vi "Window Memory write - Target.vi"(11 "Hanning window":bool=TRUE) -> ()   [LabVIEW 2014]
uses:
  <vilib>/rvi/Emulation/niFpgaGetClockAttributes.vi
  <vilib>/rvi/Emulation/niFpgaSctlEmulationGetInTimedLoop.vi
  <vilib>/rvi/Emulation/niFpgaEmulationReportErrorSimple.vi
  <vilib>/rvi/Memory/Memory_Emulation/nirvimemoryFastEmulation.vi
  <vilib>/rvi/Memory/Memory_Emulation/nirvimemoryEmulation.vi
  <vilib>/rvi/Emulation/niFpgaEmulationIsFPGAContextNoSignature.vi
  <vilib>/rvi/DataTransferAndStorage/Container/Common/niFpgaContainerGetUniqueNameForEmu.vi
  <vilib>/rvi/Emulation/niFpgaProcessEmulError.vi
  <vilib>/rvi/errors/nirviReportUnexpectedCaseInternalError (U32).vi
  <vilib>/rvi/Emulation/niFpgaCriticalErrorInLSC.vi
  <vilib>/rvi/DataTransferAndStorage/Container/XNode/niFpgaContainer.xnode
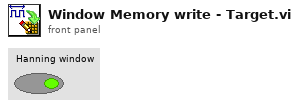
[diagram p1: front panel]
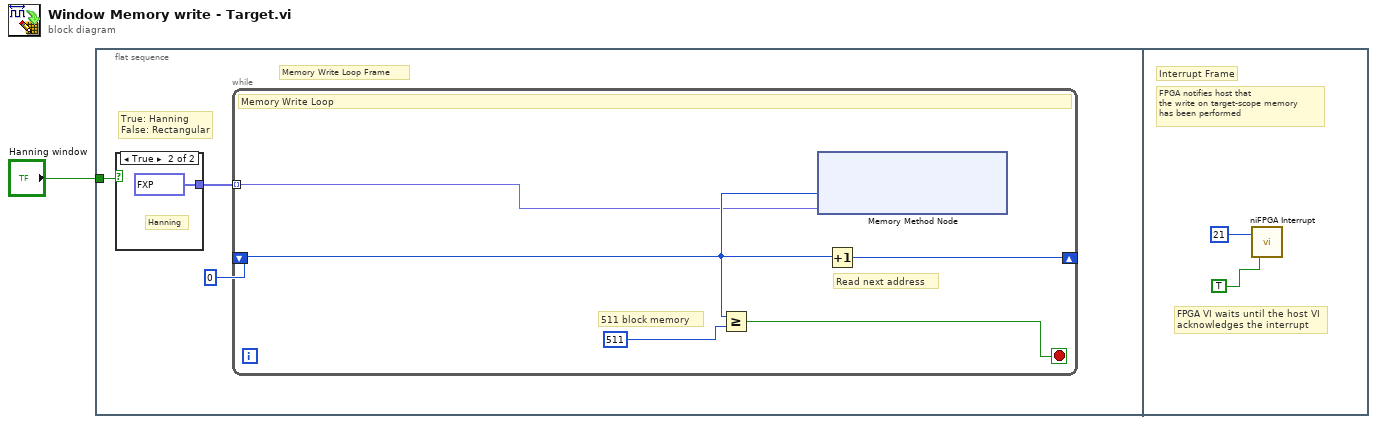
[diagram p0: block diagram]
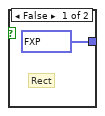
[diagram p2: hidden frame]
diagram:
  n1 = flat-sequence {
    tunnel: "Hanning window" -> [w3]
    frame #0 {
      # "True: Hanning\nFalse: Rectangular"
      # "Memory Write Loop Frame"
      n2 = case shown="True" w3 {
        tunnel: [fxp<+,8,1>[] [1.0, 1.0, 1.0, 1.0, 1.0, 1.0, 1.0, 1.0, 1.0, 1.0, 1.0, 1.0, 1.0, 1.0, 1.0, 1.0, 1.0, 1.0, 1.0, 1.0, 1.0, 1.0, 1.0, 1.0, 1.0, 1.0, 1.0, 1.0, 1.0, 1.0, 1.0, 1.0, 1.0, 1.0, 1.0, 1.0, 1.0, 1.0, 1.0, 1.0, 1.0, 1.0, 1.0, 1.0, 1.0, 1.0, 1.0, 1.0, 1.0, 1.0, 1.0, 1.0, 1.0, 1.0, 1.0, 1.0, 1.0, 1.0, 1.0, 1.0, 1.0, 1.0, 1.0, 1.0, 1.0, 1.0, 1.0, 1.0, 1.0, 1.0, 1.0, 1.0, 1.0, 1.0, 1.0, 1.0, 1.0, 1.0, 1.0, 1.0, 1.0, 1.0, 1.0, 1.0, 1.0, 1.0, 1.0, 1.0, 1.0, 1.0, 1.0, 1.0, 1.0, 1.0, 1.0, 1.0, 1.0, 1.0, 1.0, 1.0, 1.0, 1.0, 1.0, 1.0, 1.0, 1.0, 1.0, 1.0, 1.0, 1.0, 1.0, 1.0, 1.0, 1.0, 1.0, 1.0, 1.0, 1.0, 1.0, 1.0, 1.0, 1.0, 1.0, 1.0, 1.0, 1.0, 1.0, 1.0, 1.0, 1.0, 1.0, 1.0, 1.0, 1.0, 1.0, 1.0, 1.0, 1.0, 1.0, 1.0, 1.0, 1.0, 1.0, 1.0, 1.0, 1.0, 1.0, 1.0, 1.0, 1.0, 1.0, 1.0, 1.0, 1.0, 1.0, 1.0, 1.0, 1.0, 1.0, 1.0, 1.0, 1.0, 1.0, 1.0, 1.0, 1.0, 1.0, 1.0, 1.0, 1.0, 1.0, 1.0, 1.0, 1.0, 1.0, 1.0, 1.0, 1.0, 1.0, 1.0, 1.0, 1.0, 1.0, 1.0, 1.0, 1.0, 1.0, 1.0, 1.0, 1.0, 1.0, 1.0, 1.0, 1.0, 1.0, 1.0, 1.0, 1.0, 1.0, 1.0, 1.0, 1.0, 1.0, 1.0, 1.0, 1.0, 1.0, 1.0, 1.0, 1.0, 1.0, 1.0, 1.0, 1.0, 1.0, 1.0, 1.0, 1.0, 1.0, 1.0, 1.0, 1.0, 1.0, 1.0, 1.0, 1.0, 1.0, 1.0, 1.0, 1.0, 1.0, 1.0, 1.0, 1.0, 1.0, 1.0, 1.0, 1.0, 1.0, 1.0, 1.0, 1.0, 1.0, 1.0, 1.0, 1.0, 1.0, 1.0, 1.0, 1.0, 1.0, 1.0, 1.0, 1.0, 1.0, 1.0, 1.0, 1.0, 1.0, 1.0, 1.0, 1.0, 1.0, 1.0, 1.0, 1.0, 1.0, 1.0, 1.0, 1.0, 1.0, 1.0, 1.0, 1.0, 1.0, 1.0, 1.0, 1.0, 1.0, 1.0, 1.0, 1.0, 1.0, 1.0, 1.0, 1.0, 1.0, 1.0, 1.0, 1.0, 1.0, 1.0, 1.0, 1.0, 1.0, 1.0, 1.0, 1.0, 1.0, 1.0, 1.0, 1.0, 1.0, 1.0, 1.0, 1.0, 1.0, 1.0, 1.0, 1.0, 1.0, 1.0, 1.0, 1.0, 1.0, 1.0, 1.0, 1.0, 1.0, 1.0, 1.0, 1.0, 1.0, 1.0, 1.0, 1.0, 1.0, 1.0, 1.0, 1.0, 1.0, 1.0, 1.0, 1.0, 1.0, 1.0, 1.0, 1.0, 1.0, 1.0, 1.0, 1.0, 1.0, 1.0, 1.0, 1.0, 1.0, 1.0, 1.0, 1.0, 1.0, 1.0, 1.0, 1.0, 1.0, 1.0, 1.0, 1.0, 1.0, 1.0, 1.0, 1.0, 1.0, 1.0, 1.0, 1.0, 1.0, 1.0, 1.0, 1.0, 1.0, 1.0, 1.0, 1.0, 1.0, 1.0, 1.0, 1.0, 1.0, 1.0, 1.0, 1.0, 1.0, 1.0, 1.0, 1.0, 1.0, 1.0, 1.0, 1.0, 1.0, 1.0, 1.0, 1.0, 1.0, 1.0, 1.0, 1.0, 1.0, 1.0, 1.0, 1.0, 1.0, 1.0, 1.0, 1.0, 1.0, 1.0, 1.0, 1.0, 1.0, 1.0, 1.0, 1.0, 1.0, 1.0, 1.0, 1.0, 1.0, 1.0, 1.0, 1.0, 1.0, 1.0, 1.0, 1.0, 1.0, 1.0, 1.0, 1.0, 1.0, 1.0, 1.0, 1.0, 1.0, 1.0, 1.0, 1.0, 1.0, 1.0, 1.0, 1.0, 1.0, 1.0, 1.0, 1.0, 1.0, 1.0, 1.0, 1.0, 1.0, 1.0, 1.0, 1.0, 1.0, 1.0, 1.0, 1.0, 1.0, 1.0, 1.0, 1.0, 1.0, 1.0, 1.0, 1.0, 1.0, 1.0, 1.0, 1.0, 1.0, 1.0, 1.0, 1.0, 1.0, 1.0, 1.0, 1.0, 1.0, 1.0, 1.0, 1.0, 1.0, 1.0, 1.0, 1.0, 1.0, 1.0, 1.0, 1.0, 1.0, 1.0, 1.0, 1.0, 1.0, 1.0, 1.0, 1.0, 1.0, 1.0, 1.0, 1.0, 1.0, 1.0, 1.0, 1.0, 1.0, 1.0, 1.0, 1.0, 1.0, 1.0] ("Window Array") fxp<+,8,1>[] [0.0, 0.0, 0.0, 0.0, 0.0, 0.0, 0.0, 0.0, 0.0, 0.0, 0.0, 0.0078125, 0.0078125, 0.0078125, 0.0078125, 0.0078125, 0.0078125, 0.0078125, 0.015625, 0.015625, 0.015625, 0.015625, 0.015625, 0.0234375, 0.0234375, 0.0234375, 0.0234375, 0.0234375, 0.03125, 0.03125, 0.03125, 0.0390625, 0.0390625, 0.0390625, 0.0390625, 0.046875, 0.046875, 0.046875, 0.0546875, 0.0546875, 0.0625, 0.0625, 0.0625, 0.0703125, 0.0703125, 0.078125, 0.078125, 0.078125, 0.0859375, 0.0859375, 0.09375, 0.09375, 0.1015625, 0.1015625, 0.109375, 0.109375, 0.1171875, 0.1171875, 0.125, 0.125, 0.1328125, 0.1328125, 0.140625, 0.140625, 0.1484375, 0.1484375, 0.15625, 0.15625, 0.1640625, 0.171875, 0.171875, 0.1796875, 0.1796875, 0.1875, 0.1953125, 0.1953125, 0.203125, 0.2109375, 0.2109375, 0.21875, 0.21875, 0.2265625, 0.234375, 0.234375, 0.2421875, 0.25, 0.25, 0.2578125, 0.265625, 0.2734375, 0.2734375, 0.28125, 0.2890625, 0.2890625, 0.296875, 0.3046875, 0.3125, 0.3125, 0.3203125, 0.328125, 0.328125, 0.3359375, 0.34375, 0.3515625, 0.3515625, 0.359375, 0.3671875, 0.375, 0.375, 0.3828125, 0.390625, 0.3984375, 0.40625, 0.40625, 0.4140625, 0.421875, 0.4296875, 0.4296875, 0.4375, 0.4453125, 0.453125, 0.4609375, 0.4609375, 0.46875, 0.4765625, 0.484375, 0.484375, 0.4921875, 0.5, 0.5078125, 0.515625, 0.515625, 0.5234375, 0.53125, 0.5390625, 0.5390625, 0.546875, 0.5546875, 0.5625, 0.5703125, 0.5703125, 0.578125, 0.5859375, 0.59375, 0.59375, 0.6015625, 0.609375, 0.6171875, 0.625, 0.625, 0.6328125, 0.640625, 0.6484375, 0.6484375, 0.65625, 0.6640625, 0.671875, 0.671875, 0.6796875, 0.6875, 0.6875, 0.6953125, 0.703125, 0.7109375, 0.7109375, 0.71875, 0.7265625, 0.7265625, 0.734375, 0.7421875, 0.75, 0.75, 0.7578125, 0.765625, 0.765625, 0.7734375, 0.78125, 0.78125, 0.7890625, 0.7890625, 0.796875, 0.8046875, 0.8046875, 0.8125, 0.8203125, 0.8203125, 0.828125, 0.828125, 0.8359375, 0.84375, 0.84375, 0.8515625, 0.8515625, 0.859375, 0.859375, 0.8671875, 0.8671875, 0.875, 0.875, 0.8828125, 0.8828125, 0.890625, 0.890625, 0.8984375, 0.8984375, 0.90625, 0.90625, 0.9140625, 0.9140625, 0.921875, 0.921875, 0.921875, 0.9296875, 0.9296875, 0.9375, 0.9375, 0.9375, 0.9453125, 0.9453125, 0.953125, 0.953125, 0.953125, 0.9609375, 0.9609375, 0.9609375, 0.9609375, 0.96875, 0.96875, 0.96875, 0.9765625, 0.9765625, 0.9765625, 0.9765625, 0.9765625, 0.984375, 0.984375, 0.984375, 0.984375, 0.984375, 0.9921875, 0.9921875, 0.9921875, 0.9921875, 0.9921875, 0.9921875, 0.9921875, 1.0, 1.0, 1.0, 1.0, 1.0, 1.0, 1.0, 1.0, 1.0, 1.0, 1.0, 1.0, 1.0, 1.0, 1.0, 1.0, 1.0, 1.0, 1.0, 1.0, 1.0, 0.9921875, 0.9921875, 0.9921875, 0.9921875, 0.9921875, 0.9921875, 0.9921875, 0.984375, 0.984375, 0.984375, 0.984375, 0.984375, 0.9765625, 0.9765625, 0.9765625, 0.9765625, 0.9765625, 0.96875, 0.96875, 0.96875, 0.9609375, 0.9609375, 0.9609375, 0.9609375, 0.953125, 0.953125, 0.953125, 0.9453125, 0.9453125, 0.9375, 0.9375, 0.9375, 0.9296875, 0.9296875, 0.921875, 0.921875, 0.921875, 0.9140625, 0.9140625, 0.90625, 0.90625, 0.8984375, 0.8984375, 0.890625, 0.890625, 0.8828125, 0.8828125, 0.875, 0.875, 0.8671875, 0.8671875, 0.859375, 0.859375, 0.8515625, 0.8515625, 0.84375, 0.84375, 0.8359375, 0.828125, 0.828125, 0.8203125, 0.8203125, 0.8125, 0.8046875, 0.8046875, 0.796875, 0.7890625, 0.7890625, 0.78125, 0.78125, 0.7734375, 0.765625, 0.765625, 0.7578125, 0.75, 0.75, 0.7421875, 0.734375, 0.7265625, 0.7265625, 0.71875, 0.7109375, 0.7109375, 0.703125, 0.6953125, 0.6875, 0.6875, 0.6796875, 0.671875, 0.671875, 0.6640625, 0.65625, 0.6484375, 0.6484375, 0.640625, 0.6328125, 0.625, 0.625, 0.6171875, 0.609375, 0.6015625, 0.59375, 0.59375, 0.5859375, 0.578125, 0.5703125, 0.5703125, 0.5625, 0.5546875, 0.546875, 0.5390625, 0.5390625, 0.53125, 0.5234375, 0.515625, 0.515625, 0.5078125, 0.5, 0.4921875, 0.484375, 0.484375, 0.4765625, 0.46875, 0.4609375, 0.4609375, 0.453125, 0.4453125, 0.4375, 0.4296875, 0.4296875, 0.421875, 0.4140625, 0.40625, 0.40625, 0.3984375, 0.390625, 0.3828125, 0.375, 0.375, 0.3671875, 0.359375, 0.3515625, 0.3515625, 0.34375, 0.3359375, 0.328125, 0.328125, 0.3203125, 0.3125, 0.3125, 0.3046875, 0.296875, 0.2890625, 0.2890625, 0.28125, 0.2734375, 0.2734375, 0.265625, 0.2578125, 0.25, 0.25, 0.2421875, 0.234375, 0.234375, 0.2265625, 0.21875, 0.21875, 0.2109375, 0.2109375, 0.203125, 0.1953125, 0.1953125, 0.1875, 0.1796875, 0.1796875, 0.171875, 0.171875, 0.1640625, 0.15625, 0.15625, 0.1484375, 0.1484375, 0.140625, 0.140625, 0.1328125, 0.1328125, 0.125, 0.125, 0.1171875, 0.1171875, 0.109375, 0.109375, 0.1015625, 0.1015625, 0.09375, 0.09375, 0.0859375, 0.0859375, 0.078125, 0.078125, 0.078125, 0.0703125, 0.0703125, 0.0625, 0.0625, 0.0625, 0.0546875, 0.0546875, 0.046875, 0.046875, 0.046875, 0.0390625, 0.0390625, 0.0390625, 0.0390625, 0.03125, 0.03125, 0.03125, 0.0234375, 0.0234375, 0.0234375, 0.0234375, 0.0234375, 0.015625, 0.015625, 0.015625, 0.015625, 0.015625, 0.0078125, 0.0078125, 0.0078125, 0.0078125, 0.0078125, 0.0078125, 0.0078125, 0.0, 0.0, 0.0, 0.0, 0.0, 0.0, 0.0, 0.0, 0.0, 0.0] ("Window Array")] -> w2
        frame False {
          # "Rect"
        }
        frame True {
          # "Hanning"
        }
      }
      n3 = while {
        shift-right: [w9] -> _
        shift-left: u32 0 -> [w10]
        tunnel: w2 -> [w7] mode=indexing
        stop <- w11 stop-if-true
        # "Read next address"
        # "511 block memory"
        # "Memory Write Loop"
        n4 = Greater Or Equal?(x=w10, y=u32 511) -> (x >= y?=w11:bool)
        n5 = xnode ("Memory Method Node")("Address"=w10, "Data"=w7) -> ()  [unwired: 1 in, 1 out]
        n6 = Increment(x=w10) -> (x+1=w9:u32)
      }
    }
    frame #1 {
      # "FPGA VI waits until the host VI \nacknowledges the interrupt"
      # "FPGA notifies host that\nthe write on target-scope memory\nhas been performed"
      # "Interrupt Frame"
      n7 = call <vilib>:"niFPGA Interrupt.vi"("Wait Until Cleared (F)"=TRUE, "IRQ Number (0)"=u8 21) -> ()  [unwired: 1 in]
    }
  }
